vi "Write Digital Outputs.vi"(8 "error in (no error)":errorcluster, 10 "Digital Outputs":bool[](array[boolean]), 11 "VISA Refnum in":refnum<visa-resource-name>) -> (0 "error out":errorcluster, 3 "VISA resource name out":refnum<visa-resource-name>)   [LabVIEW 2024, in "CTIWrapper.lvlib"]
uses:
  CTIWrapper.lvlib
  <instrlib>/HandsOnPi2040/Public/DigOuts.ctl
  <instrlib>/HandsOnPi2040/HandsOnPi2040.lvlib
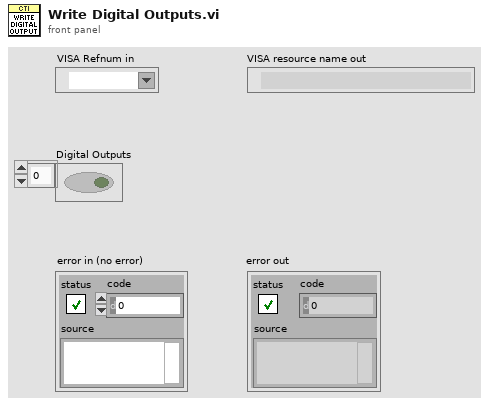
[diagram p1: front panel]
types:
  T1 = typedef "HandsOnPi2040.lvlib/DigOuts.ctl" = enum16{"No DO - Error", "DO1 (GPIO2)", "DO2 (GPIO3)", "DO3 (GPIO4)", "DO4 (GPIO5)", "BEEP (GPIO6)"}
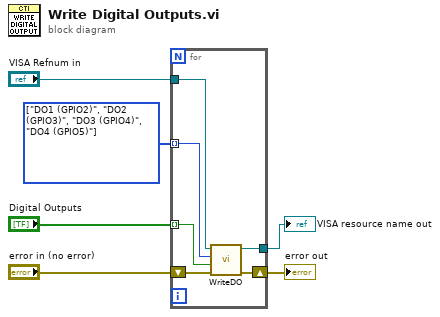
[diagram p0: block diagram]
diagram:
  w4 = T1[] [enum."DO1 (GPIO2)", enum."DO2 (GPIO3)", enum."DO3 (GPIO4)", enum."DO4 (GPIO5)"] items=["No DO - Error", "DO1 (GPIO2)", "DO2 (GPIO3)", "DO3 (GPIO4)", "DO4 (GPIO5)", "BEEP (GPIO6)"] ("Array")
  n1 = for {
    tunnel: "Digital Outputs" -> [w12] mode=indexing
    tunnel: "VISA Refnum in" -> [w11]
    tunnel: w4 -> [w10] mode=indexing
    tunnel: [w8] -> w2
    shift-right: [w9] -> w3
    shift-left: "error in (no error)" -> [w7]
    n2 = call <instrlib>:"WriteDO.vi"("error in (no error)"=w7, "DO Value (True)"=w12, "Output"=w10, "VISA resource name"=w11) -> ("error out"=w9:errorcluster, "VISA resource name out"=w8:refnum<visa-resource-name>)  [unwired: 6 in]
  }
  "error out" <- w3
  "VISA resource name out" <- w2
